vi "fgv_single-sequence.vi"(7 "cmd":T2, 8 "error in":errorcluster, 11 "Single sequence":T1) -> (0 "error out":errorcluster, 3 "queue out":refnum<queue>)   [LabVIEW 2019]
uses:
  _ctrl/create-rw-close.ctl
  Durability/sequence_single.ctl
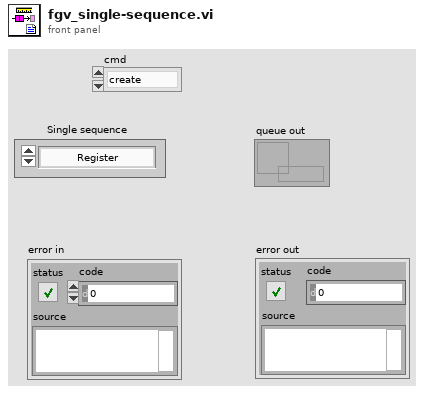
[diagram p1: front panel]
types:
  T1 = typedef "sequence_single.ctl" = enum16{"Register", "RC", "B1", "B2", "B3", "Oper_LV", "Oper_HV", "ContR_LV"}
  T2 = typedef "create-rw-close.ctl" = enum16{"create", "write", "read", "delete", "close"}
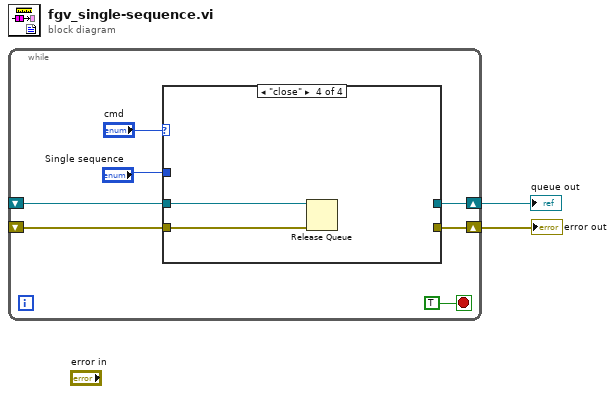
[diagram p0: block diagram]
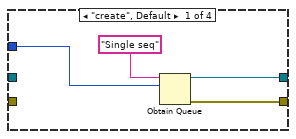
[diagram p2: hidden frame]
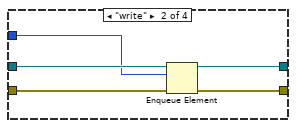
[diagram p3: hidden frame]
diagram:
  n1 = while {
    shift-right: [w7] -> w1
    shift-left: _ -> [w5]
    shift-right: [w6] -> w2
    shift-left: _ -> [w4]
    stop <- TRUE stop-if-true
    n2 = case shown="\"close\"" "cmd" {
      tunnel: [w13 w17 w19 _] -> w7
      tunnel: [w12 w15 w20 _] -> w6
      tunnel: "Single sequence" -> [w10 w14 _ _]
      tunnel: w5 -> [_ w18 w19 w21]
      tunnel: w4 -> [_ w16 w20 w22]
      frame "create", Default {
        n3 = Obtain Queue(name (unnamed)="Single seq", element data type=w10) -> (queue out=w13:refnum<queue>, error out=w12:errorcluster)  [unwired: 3 in, 1 out]
      }
      frame "write" {
        n4 = Enqueue Element(queue=w18, element=w14, error in (no error)=w16) -> (queue out=w17:refnum<queue>, error out=w15:errorcluster)  [unwired: 1 in, 1 out]
      }
      frame "read" {
      }
      frame "close" {
        n5 = Release Queue(queue=w21, error in (no error)=w22) -> ()  [unwired: 1 in, 3 out]
      }
    }
  }
  "error out" <- w2
  "queue out" <- w1
